vi "数据处理直接插入整合 (子VI).vi"   [LabVIEW 2016, in "数据传输系统.lvlib"]
types:
  T1 = cluster{"PH":string[][], "CODCr":string[][], "氨氮":string[][], "CODMn":string[][], "总氮":string[][], "总磷":string[][], "电导率":string[][], "水温":string[][], "DO":string[][], "浊度":string[][], "叶绿素":string[][], "藻密度":string[][], "DOper":string[][], "盐度":string[][], "水位":string[][], "流速":string[][], "瞬时流量":string[][], "累计流量":string[][]}
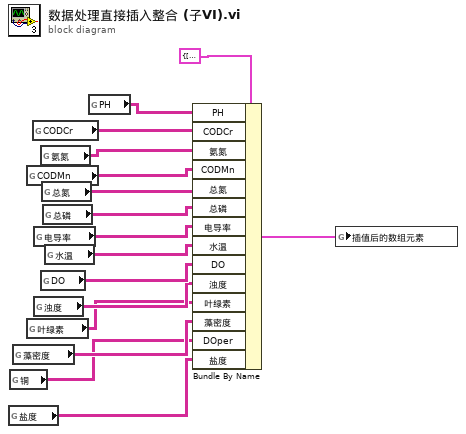
[diagram p0: block diagram]
diagram:
  n1 = global read "全局 所有参数.vi" "盐度"() -> (w1:string[][])
  n2 = global read "全局 所有参数.vi" "铜"() -> (w2:string[][])
  n3 = global read "全局 所有参数.vi" "藻密度"() -> (w3:string[][])
  n4 = global read "全局 所有参数.vi" "CODMn"() -> (w11:string[][])
  n5 = global read "全局 所有参数.vi" "叶绿素"() -> (w4:string[][])
  n6 = global read "全局 所有参数.vi" "CODCr"() -> (w13:string[][])
  n7 = global read "全局 所有参数.vi" "电导率"() -> (w8:string[][])
  n8 = global read "全局 所有参数.vi" "浊度"() -> (w5:string[][])
  n9 = global read "全局 所有参数.vi" "氨氮"() -> (w12:string[][])
  n10 = global read "全局 所有参数.vi" "DO"() -> (w6:string[][])
  n11 = global read "全局 所有参数.vi" "总氮"() -> (w10:string[][])
  n12 = global read "全局 所有参数.vi" "总磷"() -> (w9:string[][])
  n13 = global read "全局 所有参数.vi" "水温"() -> (w7:string[][])
  n14 = global read "全局 所有参数.vi" "PH"() -> (w14:string[][])
  n15 = Bundle By Name(cluster=T1 {"PH"=[], "CODCr"=[], "氨氮"=[], "CODMn"=[], "总氮"=[], "总磷"=[], "电导率"=[], "水温"=[], "DO"=[], "浊度"=[], "叶绿素"=[], "藻密度"=[], "DOper"=[], "盐度"=[], "水位"=[], "流速"=[], "瞬时流量"=[], "累计流量"=[]} ("插值后的数组元素"), "PH"=w14, "CODCr"=w13, "氨氮"=w12, "CODMn"=w11, "总氮"=w10, "总磷"=w9, "电导率"=w8, "水温"=w7, "DO"=w6, "浊度"=w5, "叶绿素"=w4, "藻密度"=w3, "DOper"=w2, "盐度"=w1) -> (w15:T1)
  n16 = global write "插值后的新数组.vi" "插值后的数组元素"(w15) -> ()
